vi "Get Group Direction.vi"(8 "error in (no error)":errorcluster, 11 "Item Ref in":T2 format="%.0x") -> (0 "error out":errorcluster, 1 "found?":bool, 2 "direction":T1, 3 "Item Ref out":T2 format="%.0x")   [LabVIEW 2020, in "DSF System Explorer.lvlib"]
uses:
  DSF System Explorer.lvlib
  <vilib>/NI VeriStand/Custom Device API/Custom Device Item Ref.ctl
  Includes/DSF Core.lvlibp/Typedefs/DSF Direction.ctl
  Shared/Group Page GUID.vi
  <vilib>/NI VeriStand/Custom Device API/Custom Device API.lvlib
  Shared/DSF Shared.lvlib
  Includes/DSF Core.lvlibp
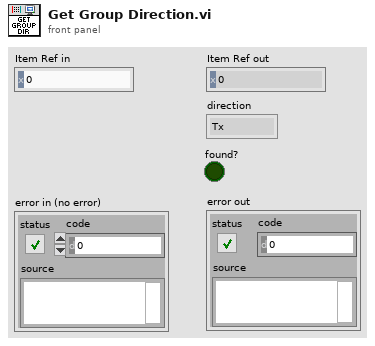
[diagram p1: front panel]
types:
  T1 = typedef "DSF Core.lvlibp/DSF Direction.ctl" = enum8{"Tx", "Rx"}
  T2 = typedef "Custom Device API.lvlib/Custom Device Item Ref.ctl" = u64
  T3 = typedef "Custom Device API.lvlib/Custom Device Item Info.ctl" = cluster{"Name":string, "Is Channel":bool, "GUID":string, "Is Waveform":bool}
  T4 = typedef "DSF Core.lvlibp/Group Configuration.lvclass/Core Group Configuration.ctl" = cluster{"name":string, "direction":T1, "cycle timing":T5, "timeout behavior":T6, "enable conversion":bool}
  T5 = typedef "DSF Core.lvlibp/DSF Timing Info.ctl" = cluster{"priority":u64, "decimation":u64, "offset":u64}
  T6 = typedef "DSF Core.lvlibp/DSF Timeout Behavior.ctl" = enum8{"Increment Late Count", "Throw Error"}
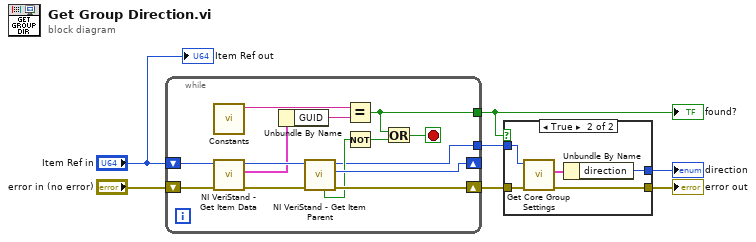
[diagram p0: block diagram]
diagram:
  n1 = while {
    shift-right: [w15] -> w3
    shift-left: "error in (no error)" -> [w18]
    shift-right: [w14] -> _
    shift-left: "Item Ref in" -> [w19]
    tunnel: [w11] -> w4
    tunnel: [w8] -> w5
    stop <- w9 stop-if-true
    n2 = call-poly "Constants.vi"() -> ("Group GUID"=w21:string)  [unwired: 11 in]
    n3 = call <vilib>:"NI VeriStand - Get Item Data.vi"("error in (no error)"=w18, "Item Ref in"=w19) -> ("error out"=w13:errorcluster, "Item Info"=w16:T3, "Item Ref out"=w17:T2)  [unwired: 6 in, 1 out]
    n4 = Unbundle By Name(w16) -> ("GUID"=w20:string)
    n5 = call <vilib>:"NI VeriStand - Get Item Parent.vi"("error in (no error)"=w13, "Item Ref in"=w17) -> ("error out"=w15:errorcluster, "Parent Ref"=w14:T2, "Item Ref out"=w11:T2, "Found"=w12:bool)  [unwired: 6 in]
    n6 = Equal?(x=w21, y=w20) -> (x = y?=w8:bool)
    n7 = Not(x=w12) -> (.not. x?=w10:bool)
    n8 = Or(x=w8, y=w10) -> (x .or. y?=w9:bool)
  }
  "found?" <- w5
  n9 = case shown="True" w5 {
    tunnel: w4 -> [_ w26]
    tunnel: w3 -> [w22 w27]
    tunnel: [w22 w25] -> w2
    tunnel: [_ w23] -> w1
    frame False {
    }
    frame True {
      n10 = call "Get Core Group Settings.vi"("error in (no error)"=w27, "Item Ref in"=w26) -> ("error out"=w25:errorcluster, "group configuration"=w24:T4)  [unwired: 7 in, 1 out]
      n11 = Unbundle By Name(w24) -> ("direction"=w23:T1)
    }
  }
  "error out" <- w2
  "direction" <- w1
  "Item Ref out" <- "Item Ref in"
